vi "Fix HTTPS Url.vi"() -> ()   [LabVIEW 2020, in "GPackScratch.lvlib"]
uses:
  GPackScratch.lvlib
  <vilib>/regexp/Match Regular Expression.xnode
panel:
  out "String":string
  in  "string":string
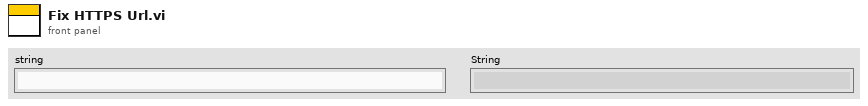
[diagram p1: front panel]
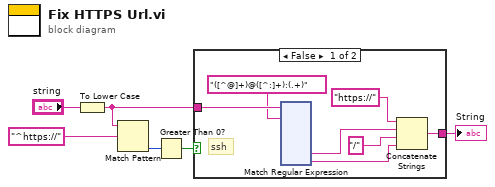
[diagram p0: block diagram]
diagram:
  n1 = To Lower Case(string="string") -> (all lower case string=w3:string)
  n2 = Match Pattern(string=w3, regular expression="^https://") -> (offset past match=w5:i32)  [unwired: 1 in, 3 out]
  n3 = Greater Than 0?(x=w5) -> (x > 0?=w4:bool)
  n4 = case shown="False" w4 {
    tunnel: w3 -> [w13 w132]
    tunnel: [w7 w132] -> w1
    frame False {
      # "ssh"
      n5 = xnode "Match Regular Expression"("input string"=w13, "regular expression"="([^@]+)@([^:]+):(.+)") -> ("submatch 2"=w10:string, "submatch 3"=w8:string)  [unwired: 4 in, 6 out]
      n6 = Concatenate Strings("https://" ("string"), w10, "/" ("string"), w8) -> (w7:string)
    }
    frame True {
      # "https"
    }
  }
  "String" <- w1
